vi "Loop Counter.vi"(3 "Time to Wait A":u8) -> (1 "Time Expired A":bool)   [LabVIEW 2014]
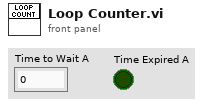
[diagram p1: front panel]
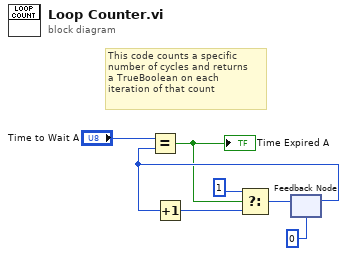
[diagram p0: block diagram]
diagram:
  # "This code counts a specific \nnumber of cycles and returns \na TrueBoolean on each\niteration of that count"
  n1 = feedback #1(u8 0) -> (w5:u8)
  n2 = Equal?(x="Time to Wait A", y=w5) -> (x = y?=w1:bool)
  "Time Expired A" <- w1
  n3 = Increment(x=w5) -> (x+1=w2:u8)
  n4 = Select(t=u8 1 ("f"), s=w1, f=w2) -> (s? t:f=w6:u8)
  n5 = feedback-in #1(w6) -> ()
